vi "ATS9350_NPT_on-FPGA_FFT_Float.vi"() -> ()   [LabVIEW 2018]
panel:
  out "Graph":sgl[](graph)
  in  "stop":bool
  # "Connect proper signal to channel A before starting acquisition\n(e.g. 1Vpp 1kHz sine wave)"
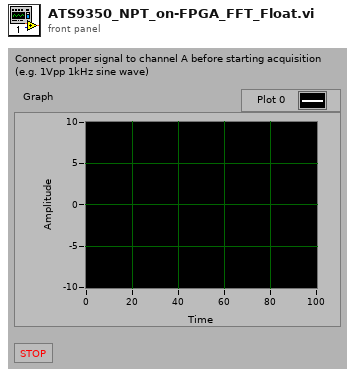
[diagram p1: front panel]
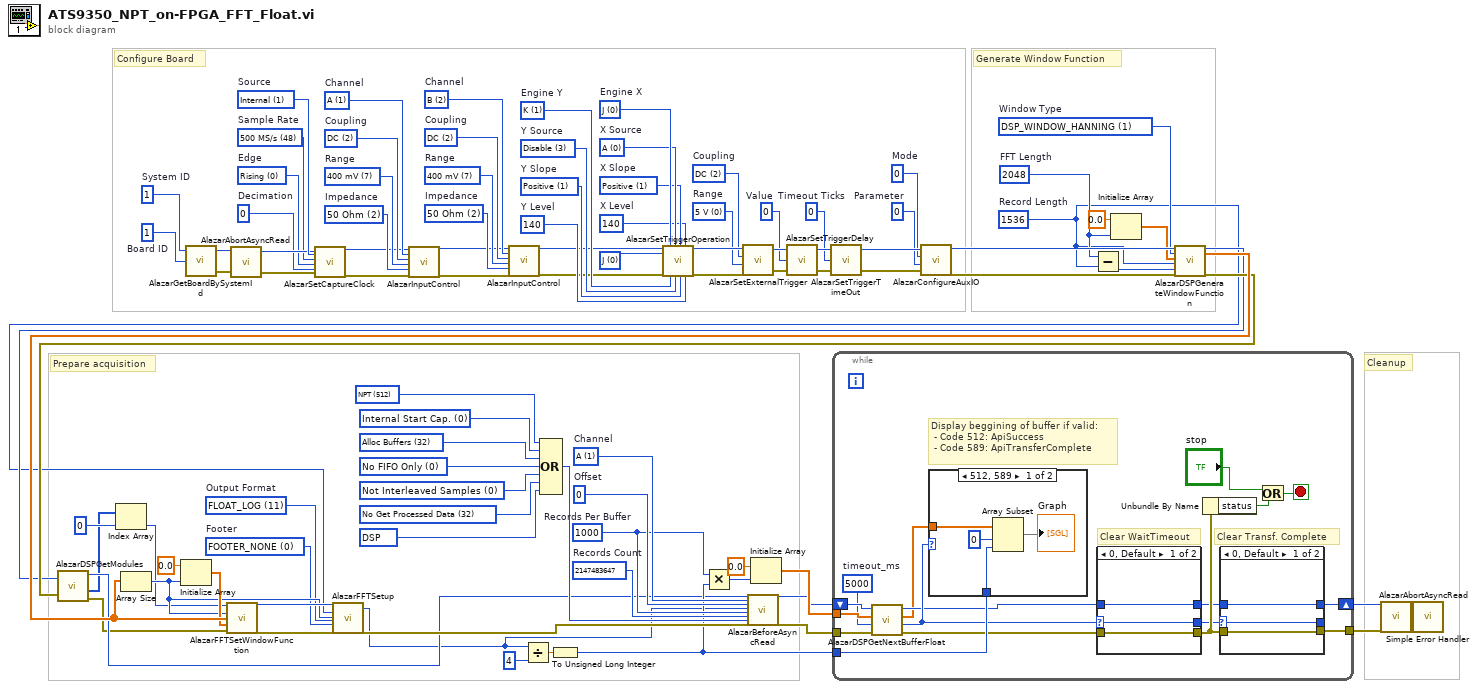
[diagram p0: block diagram]
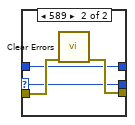
[diagram p3: hidden frame]
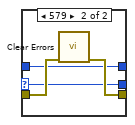
[diagram p4: hidden frame]
diagram:
  w14 = u32 11 items=["FLOAT_AMP2"=10, "FLOAT_LOG"=11]  # Output Format
  w13 = u32 0 items=["FOOTER_NONE", "FOOTER_NPT"]  # Footer
  w27 = u32 2048  # FFT Length
  w25 = u32 1 items=["DSP_WINDOW_NONE", "DSP_WINDOW_HANNING", "DSP_WINDOW_HAMMING", "DSP_WINDOW_BLACKMAN", "DSP_WINDOW_BLACKMAN_HARRIS", "DSP_WINDOW_BARTLETT"]  # Window Type
  w1 = u32 1536  # Record Length
  w31 = u32 16384 items=["DSP"=16384]
  w61 = u32 2 items=["50 Ohm"=2]  # Impedance
  w60 = u32 7 items=["400 mV"=7]  # Range
  w62 = u32 2 items=["DC"=2]  # Coupling
  w63 = u8 2 items=["A"=1, "B"=2, "C"=4, "D"=8]  # Channel
  w39 = u32 0  # Parameter
  w38 = u32 0  # Mode
  w37 = u32 0  # Timeout Ticks
  w44 = u32 0  # Value
  w48 = u32 0 items=["5 V", "1 V", "TTL"]  # Range
  w47 = u32 2 items=["AC"=1, "DC"=2]  # Coupling
  w51 = u32 140  # Y Level
  w52 = u32 1 items=["Positive"=1, "Negative"=2]  # Y Slope
  w53 = u32 3 items=["A", "B", "External", "Disable", "C", "D"]  # Y Source
  w55 = u32 140  # X Level
  w56 = u32 1 items=["Positive"=1, "Negative"=2]  # X Slope
  w57 = u32 0 items=["A", "B", "External", "Disable", "C", "D"]  # X Source
  w54 = u32 1 items=["J", "K"]  # Engine Y
  w58 = u32 0 items=["J", "K"]  # Engine X
  w59 = u32 0 items=["J", "K", "J OR K", "J AND K", "J XOR K", "J AND NOT K", "NOT J AND K"] ("Op.")
  w66 = u32 2 items=["50 Ohm"=2]  # Impedance
  w67 = u32 7 items=["400 mV"=7]  # Range
  w68 = u32 2 items=["DC"=2]  # Coupling
  w69 = u8 1 items=["A"=1, "B"=2, "C"=4, "D"=8]  # Channel
  w71 = u32 0  # Decimation
  w72 = u32 0 items=["Rising", "Falling"]  # Edge
  w73 = u32 48 items=["1 kS/s"=1, "2 kS/s"=2, "5 kS/s"=4, "10 kS/s"=8, "20 kS/s"=10, "50 kS/s"=12, "100 kS/s"=14, "200 kS/s"=16, "500 kS/s"=18, "1 MS/s"=20, "2 MS/s"=24, "5 MS/s"=26, "10 MS/s"=28, "20 MS/s"=30, "50 MS/s"=34, "100 MS/s"=36, "125 MS/s"=37, "200 MS/s"=40, "500 MS/s"=48, "800 MS/s"=50, "1000 MS/s"=53, "1200 MS/s"=55, "1500 MS/s"=58, "1800 MS/s"=61, "USER_DEF"=0]  # Sample Rate
  w75 = u32 1 items=["Internal"=1, "Fast External"=2, "Medium External"=3, "Slow External"=4, "External AC"=5, "External DC"=6, "External 10MHz"=7]  # Source
  w79 = u32 1  # Board ID
  w78 = u32 1  # System ID
  w87 = u32 2147483647  # Records Count
  w12 = u32 1000  # Records Per Buffer
  w88 = u32 0  # Offset
  w32 = u32 1 items=["A"=1]  # Channel
  w95 = u32 32 items=["No Get Processed Data"=32, "Get Processed Data"=8192]
  w94 = u32 0 items=["Not Interleaved Samples"=0, "Interleave Samples"=4096]
  w90 = u32 0 items=["No FIFO Only"=0, "FIFO Only"=2048]
  w93 = u32 32 items=["Alloc Buffers"=32]
  w92 = u32 0 items=["Internal Start Cap.", "External Start Cap."]
  w91 = u32 512 items=["Traditional"=0, "NPT"=512, "Continuous"=256, "Triggered Streaming"=1024]
  # "Generate Window Function"
  # "Configure Board"
  # "Cleanup"
  # "Prepare acquisition"
  n1 = call "AlazarGetBoardBySystemId.vi"("Board ID"=w79, "System ID"=w78) -> ("error out"=w76:errorcluster, "Handle"=w77:u64)  [unwired: 1 in, 1 out]
  n2 = call "AlazarAbortAsyncRead.vi"("Handle"=w77, "error in (no error)"=w76) -> ("Handle"=w74:u64, "error out"=w70:errorcluster)  [unwired: 1 out]
  n3 = call "AlazarSetCaptureClock.vi"("Handle"=w74, "Source"=w75, "Sample Rate"=w73, "Edge"=w72, "Decimation"=w71, "error in (no error)"=w70) -> ("Handle"=w65:u64, "error out"=w64:errorcluster)  [unwired: 11 in, 1 out]
  n4 = call "AlazarInputControl.vi"("Handle"=w65, "Channel"=w69, "Coupling"=w68, "Range"=w67, "Impedance"=w66, "error in (no error)"=w64) -> ("Handle"=w33:u64, "error out"=w36:errorcluster)  [unwired: 11 in, 1 out]
  n5 = call "AlazarInputControl.vi"("Handle"=w33, "Channel"=w63, "Coupling"=w62, "Range"=w60, "Impedance"=w61, "error in (no error)"=w36) -> ("Handle"=w34:u64, "error out"=w35:errorcluster)  [unwired: 11 in, 1 out]
  n6 = Compound Arithmetic op=OR(w91, w92, w93, w90, w94, w95, w31) -> (w89:u32)
  n7 = call "AlazarSetTriggerOperation.vi"("Handle"=w34, "Trigger Operation"=w59, "error in (no error)"=w35, "Trigger Engine 1"=w58, "Trigger Engine 2"=w54, "Source 1"=w57, "Source 2"=w53, "Slope 1"=w56, "Slope 2"=w52, "Level 1"=w55, "Level 2"=w51) -> ("Handle"=w50:u64, "error out"=w49:errorcluster)  [unwired: 6 in, 1 out]
  n8 = call "AlazarSetExternalTrigger.vi"("error in (no error)"=w49, "Range ID"=w48, "Coupling ID"=w47, "Handle"=w50) -> ("error out"=w45:errorcluster, "Handle"=w46:u64)  [unwired: 1 out]
  n9 = call "AlazarSetTriggerDelay.vi"("error in (no error)"=w45, "Delay"=w44, "Handle"=w46) -> ("error out"=w42:errorcluster, "Handle"=w43:u64)  [unwired: 1 out]
  n10 = call "AlazarSetTriggerTimeOut.vi"("error in (no error)"=w42, "Timeout Ticks"=w37, "Handle"=w43) -> ("error out"=w40:errorcluster, "Handle"=w41:u64)  [unwired: 1 out]
  n11 = call "AlazarConfigureAuxIO.vi"("error in (no error)"=w40, "Parameter"=w39, "Mode"=w38, "Handle"=w41) -> ("error out"=w29:errorcluster, "Handle"=w30:u64)  [unwired: 1 out]
  n12 = Subtract(x=w27, y=w1) -> (x-y=w24:u32)
  n13 = Initialize Array(sgl 0.0, w27) -> (w26:sgl[])
  n14 = call "AlazarDSPGenerateWindowFunction.vi"("Handle"=w30, "Window Type"=w25, "window"=w26, "WindowLength_samples"=w1, "PaddingLength_samples"=w24, "error in (no error)"=w29) -> ("Handle"=w8:u64, "window"=w23:sgl[], "error out"=w9:errorcluster)  [unwired: 10 in, 1 out]
  n15 = call "AlazarDSPGetModules.vi"("Handle"=w8, "error in (no error)"=w9) -> ("Handle"=w7:u64, "DSP Modules"=w4:u64[], "error out"=w6:errorcluster)  [unwired: 1 out]
  n16 = Index Array(array=w4, index=u32 0) -> (element=w3:u64)
  n17 = Array Size(array=w23) -> (size(s)=w15:i32)
  n18 = Initialize Array(sgl 0.0, w15) -> (w21:sgl[])
  n19 = call "AlazarFFTSetWindowFunction.vi"("DSP Handle"=w3, "Samples per record"=w15, "Real window array"=w23, "Imag window array"=w21, "error in (no error)"=w6) -> ("DSP Handle"=w20:u64, "error out"=w19:errorcluster)  [unwired: 9 in]
  n20 = call "AlazarFFTSetup.vi"("DSP Handle"=w20, "Record Length (samples)"=w1, "FFT Length (samples)"=w15, "Output Format"=w14, "Footer"=w13, "error in (no error)"=w19) -> ("Bytes Per Output Record"=w2:u32, "error out"=w18:errorcluster)  [unwired: 18 in, 2 out]
  n21 = Divide(x=w2, y=4) -> (x/y=w16:dbl)
  n22 = To Unsigned Long Integer(number=w16) -> (unsigned 32bit integer=w10:u32)
  n23 = Multiply(x=w12, y=w10) -> (x*y=w11:u32)
  n24 = call "AlazarBeforeAsyncRead.vi"("Handle"=w7, "Channel Select"=w32, "Transfer Offset"=w88, "Transfer Length"=w2, "Records Per Buffer"=w12, "Records Per Acquisition"=w87, "Flags"=w89, "error in (no error)"=w18) -> ("Handle"=w84:u64, "error out"=w83:errorcluster)  [unwired: 17 in, 1 out]
  n25 = Initialize Array(sgl 0.0, w11) -> (w85:sgl[])
  n26 = while {
    tunnel: w85 -> [w102]
    tunnel: w83 -> [w100]
    tunnel: [w105] -> w80
    shift-right: [w106] -> w81
    shift-left: w84 -> [w103]
    tunnel: w10 -> [w104]
    stop <- w109 stop-if-true
    w101 = u32 5000  # timeout_ms
    # "Display beggining of buffer if valid:\n - Code 512: ApiSuccess\n - Code 589: ApiTransferComplete"
    # "Clear Transf. Complete"
    # "Clear WaitTimeout"
    n27 = call "AlazarDSPGetNextBufferFloat.vi"("error in (no error)"=w100, "timeout_ms"=w101, "Buffer"=w102, "Handle"=w103) -> ("error out"=w99:errorcluster, "Return Code"=w98:u32, "Buffer"=w96:sgl[], "Handle"=w97:u64)
    n28 = case shown="512, 589" w98 {
      tunnel: w96 -> [w114 _]
      tunnel: w104 -> [w113 _]
      frame 512, 589 {
        n29 = Array Subset(array=w114, index=0, length=w113) -> (→"Graph":sgl[])
      }
      frame Default {
      }
    }
    n30 = case shown="0, Default" w98 {
      selector: w98 -> [w125 w127]
      tunnel: w99 -> [w124 w130]
      tunnel: [w124 w129] -> w112
      tunnel: [w126 w128] -> w111
      tunnel: w97 -> [w126 w128]
      tunnel: [w125 w127] -> w110
      frame 0, Default {
      }
      frame 579 {
        n31 = call <vilib>:"Clear Errors.vi"("error in (no error)"=w130) -> ("error out"=w129:errorcluster)  [unwired: 5 in, 1 out]
      }
    }
    n32 = Unbundle By Name(w112) -> ("status"=w107:bool)
    n33 = case shown="0, Default" w110 {
      selector: w110 -> [w118 w120]
      tunnel: w112 -> [w117 w123]
      tunnel: [w117 w122] -> w105
      tunnel: [w119 w121] -> w106
      tunnel: w111 -> [w119 w121]
      tunnel: [w118 w120] -> _
      frame 0, Default {
      }
      frame 589 {
        n34 = call <vilib>:"Clear Errors.vi"("error in (no error)"=w123) -> ("error out"=w122:errorcluster)  [unwired: 5 in, 1 out]
      }
    }
    n35 = Or(x="stop", y=w107) -> (x .or. y?=w109:bool)
  }
  n36 = call "AlazarAbortAsyncRead.vi"("Handle"=w81, "error in (no error)"=w80) -> ("error out"=w82:errorcluster)  [unwired: 2 out]
  n37 = call <vilib>:"Simple Error Handler.vi"("error in (no error)"=w82) -> ()  [unwired: 4 in, 5 out]
